vi "Partial Cluster With Array Of Digital Waveform.vi"(8 "LV Control Name Paths":string[](array[string]), 9 "TS Variable Name Paths":string[](array[string]), 10 "Sequence Context":refnum<k7>, 11 "Cluster":T1={"Numeric"=0.0, "Array"=[{"t0"=timestamp(0 s since 1904-01-01), "dt"=0.0, "Y"={"transitions"=[], "data"=[]}}]}) -> (0 "error out":errorcluster, 1 "Report Text":string, 2 "PASS/FAIL Flag":bool, 3 "Cluster 2":T1)   [LabVIEW 2013]
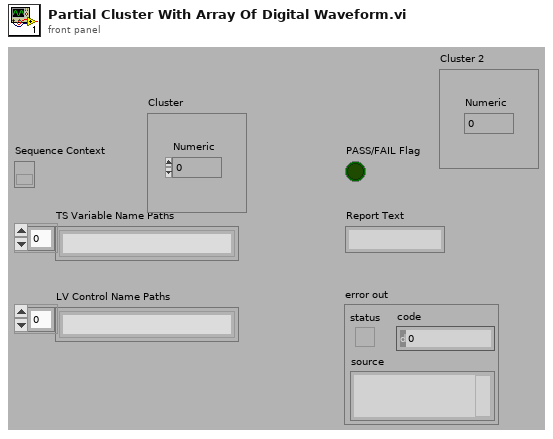
[diagram p1: front panel]
types:
  T1 = cluster{"Numeric":dbl, "Array":digitalwaveform[]}
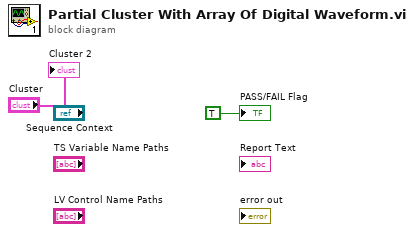
[diagram p0: block diagram]
diagram:
  "PASS/FAIL Flag" <- TRUE ("PASS/FAIL Flag")
  "Cluster 2" <- "Cluster"
